vi "X10468 SLM Make Zernike Modes.vi"(0 "R Array":dbl[][](array[numeric]), 7 "Theta Array":dbl[][](array[numeric]), 11 "Number of Modes":i32) -> (8 "Zernike Array":dbl[][][](array[numeric]))   [LabVIEW 2018]
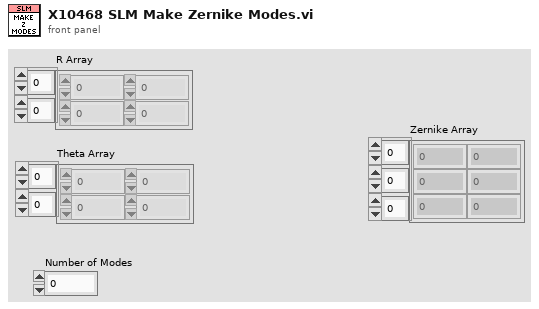
[diagram p1: front panel]
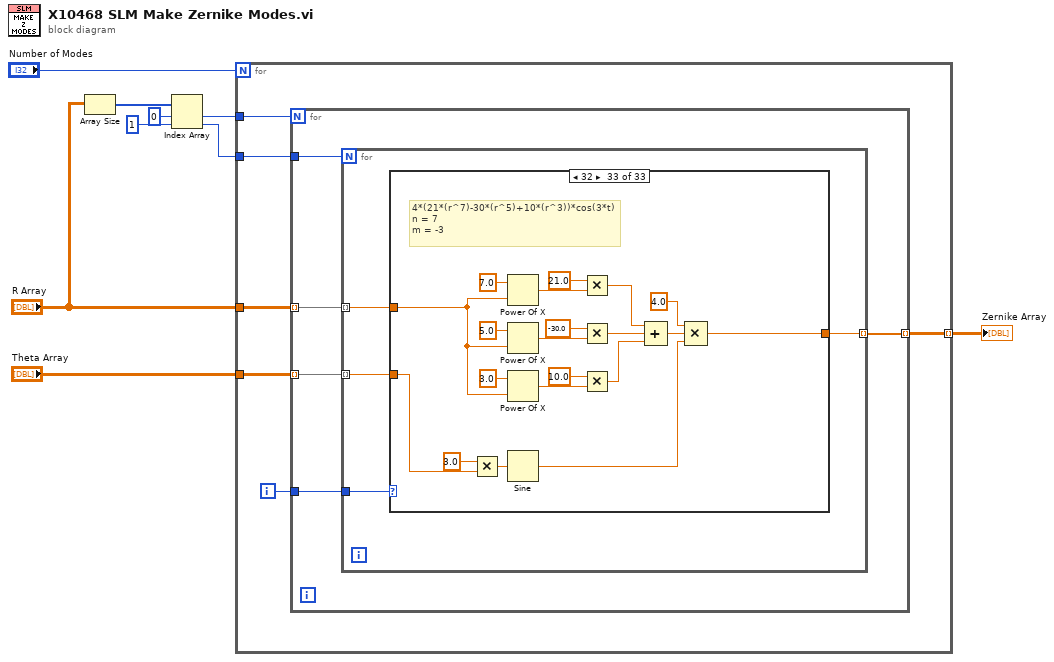
[diagram p0: block diagram]
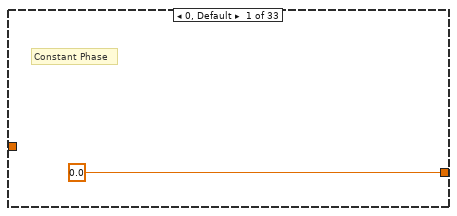
[diagram p2: hidden frame]
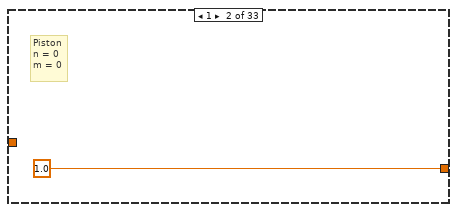
[diagram p3: hidden frame]
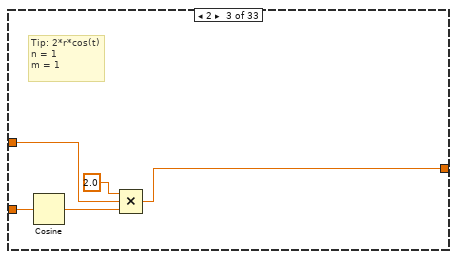
[diagram p4: hidden frame]
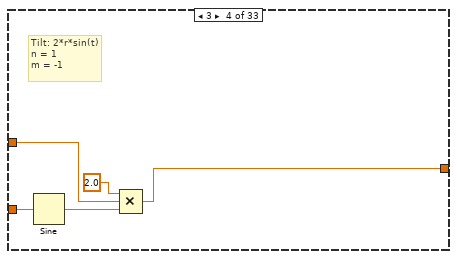
[diagram p5: hidden frame]
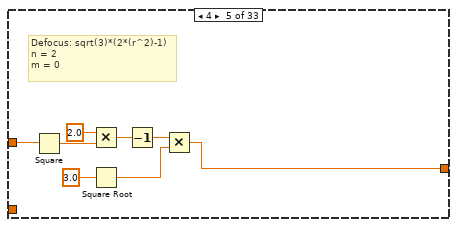
[diagram p6: hidden frame]
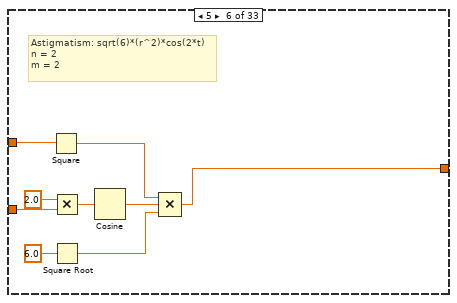
[diagram p7: hidden frame]
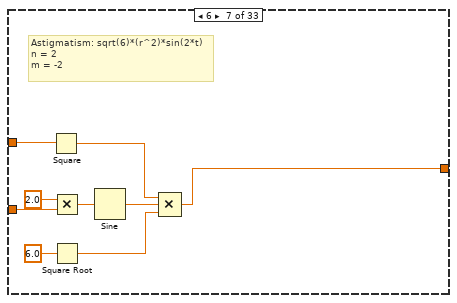
[diagram p8: hidden frame]
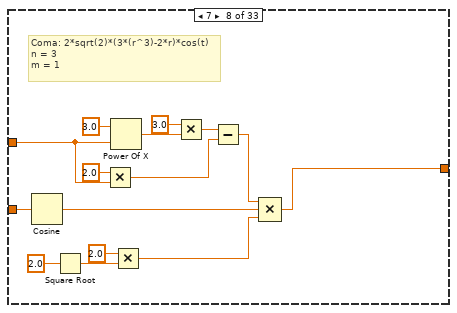
[diagram p9: hidden frame]
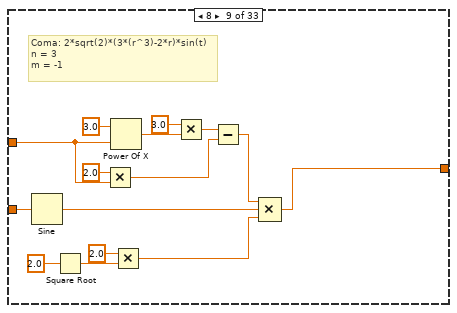
[diagram p10: hidden frame]
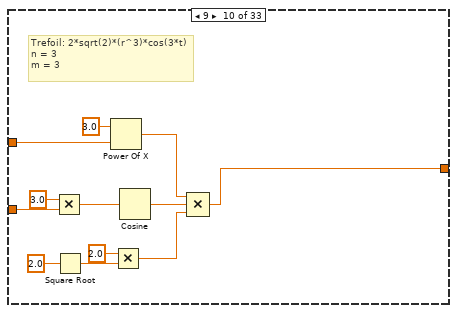
[diagram p11: hidden frame]
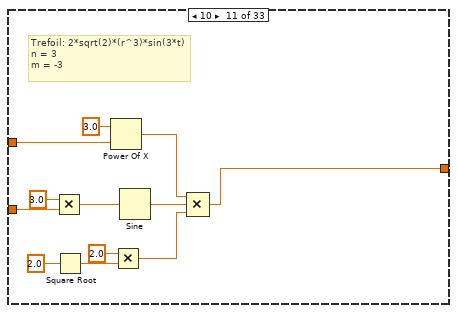
[diagram p12: hidden frame]
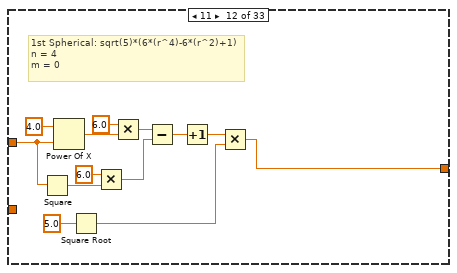
[diagram p13: hidden frame]
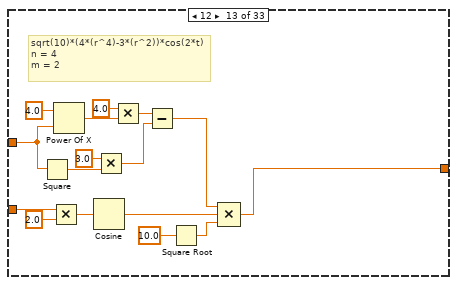
[diagram p14: hidden frame]
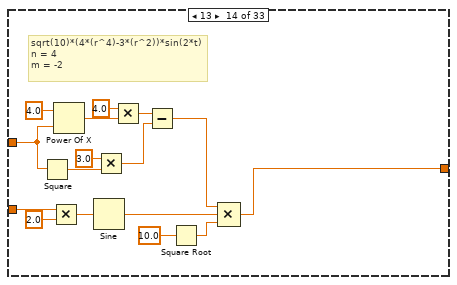
[diagram p15: hidden frame]
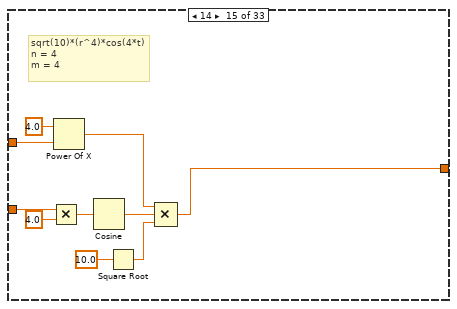
[diagram p16: hidden frame]
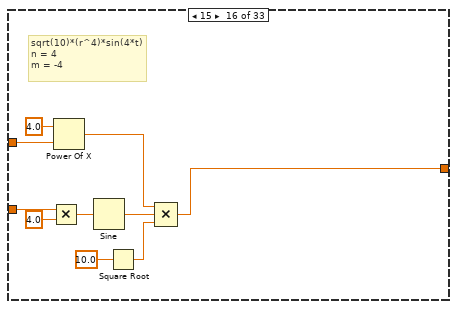
[diagram p17: hidden frame]
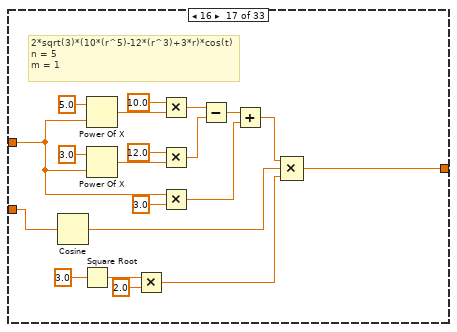
[diagram p18: hidden frame]
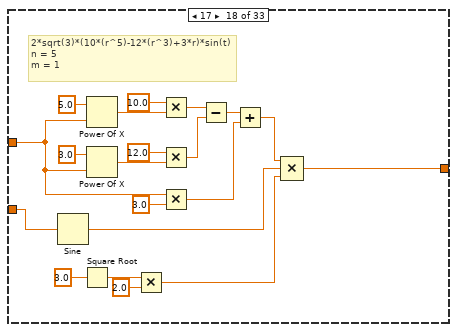
[diagram p19: hidden frame]
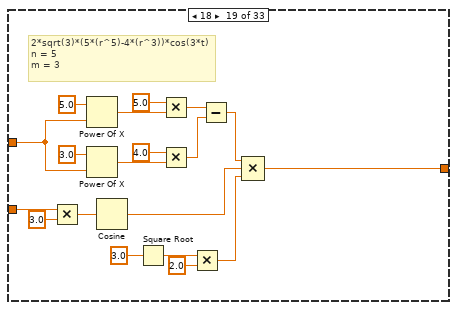
[diagram p20: hidden frame]
diagram:
  n1 = Array Size(array="R Array") -> (size(s)=w8:i32[])
  n2 = Index Array(array=w8, index #1=0 ("index"), index #2=1 ("index")) -> (element #1=w3:i32, element #2=w2:i32)
  n3 = for {
    N: "Number of Modes" -> [_]
    tunnel: "R Array" -> [w11]
    tunnel: "Theta Array" -> [w10]
    tunnel: w3 -> [w15]
    tunnel: w2 -> [w14]
    tunnel: [w12] -> w1 mode=indexing
    i -> [w13]
    n4 = for {
      N: w15 -> [_]
      tunnel: w14 -> [w20]
      tunnel: w13 -> [w19]
      tunnel: [w18] -> w12 mode=indexing
      tunnel: w11 -> [w17] mode=indexing
      tunnel: w10 -> [w16] mode=indexing
      n5 = for {
        N: w20 -> [_]
        tunnel: w19 -> [w24]
        tunnel: [w23] -> w18 mode=indexing
        tunnel: w17 -> [w22] mode=indexing
        tunnel: w16 -> [w21] mode=indexing
        n6 = case shown="32" w24 {
          tunnel: [0.0 1.0 w27 w32 w37 w47 w56 w63 w78 w97 w109 w117 w131 w147 w164 w174 w184 w204 w228 w247 w266 w278 w285 w307 w332 w349 w366 w383 w393 w410 w430 w450 w470] -> w23
          tunnel: w22 -> [_ _ w29 w34 w43 w52 w61 w71 w86 w100 w112 w124 w140 w156 w169 w179 w187 w207 w229 w248 w267 w279 w290 w311 w334 w350 w367 w384 w394 w402 w422 w444 w464]
          tunnel: w21 -> [_ _ w31 w36 _ w51 w60 w76 w91 w95 w107 _ w136 w152 w168 w178 w192 w212 w224 w243 w262 w274 _ w305 w330 w347 w364 w381 w391 w404 w424 w437 w457]
          frame 0, Default {
            # "Constant Phase"
          }
          frame 1 {
            # "Piston\nn = 0\nm = 0"
          }
          frame 2 {
            # "Tip: 2*r*cos(t)\nn = 1\nm = 1"
            n7 = Cosine(x=w31) -> (cos(x)=w30:dbl)
            n8 = Compound Arithmetic op=MULTIPLY(2.0 ("x"), w29, w30) -> (w27:dbl)
          }
          frame 3 {
            # "Tilt: 2*r*sin(t)\nn = 1\nm = -1"
            n9 = Sine(x=w36) -> (sin(x)=w35:dbl)
            n10 = Compound Arithmetic op=MULTIPLY(2.0 ("x"), w34, w35) -> (w32:dbl)
          }
          frame 4 {
            # "Defocus: sqrt(3)*(2*(r^2)-1)\nn = 2\nm = 0"
            n11 = Square(x=w43) -> (x^2=w42:dbl)
            n12 = Multiply(x=2.0, y=w42) -> (x*y=w40:dbl)
            n13 = Square Root(x=3.0) -> (sqrt(x)=w38:dbl)
            n14 = Decrement(x=w40) -> (x-1=w39:dbl)
            n15 = Multiply(x=w39, y=w38) -> (x*y=w37:dbl)
          }
          frame 5 {
            # "Astigmatism: sqrt(6)*(r^2)*cos(2*t)\nn = 2\nm = 2"
            n16 = Square(x=w52) -> (x^2=w48:dbl)
            n17 = Multiply(x=2.0, y=w51) -> (x*y=w49:dbl)
            n18 = Square Root(x=6.0) -> (sqrt(x)=w45:dbl)
            n19 = Cosine(x=w49) -> (cos(x)=w46:dbl)
            n20 = Compound Arithmetic op=MULTIPLY(w48, w46, w45) -> (w47:dbl)
          }
          frame 6 {
            # "Astigmatism: sqrt(6)*(r^2)*sin(2*t)\nn = 2\nm = -2"
            n21 = Square(x=w61) -> (x^2=w57:dbl)
            n22 = Multiply(x=2.0, y=w60) -> (x*y=w58:dbl)
            n23 = Square Root(x=6.0) -> (sqrt(x)=w54:dbl)
            n24 = Sine(x=w58) -> (sin(x)=w55:dbl)
            n25 = Compound Arithmetic op=MULTIPLY(w57, w55, w54) -> (w56:dbl)
          }
          frame 7 {
            # "Coma: 2*sqrt(2)*(3*(r^3)-2*r)*cos(t)\nn = 3\nm = 1"
            n26 = Cosine(x=w76) -> (cos(x)=w65:dbl)
            n27 = Square Root(x=2.0) -> (sqrt(x)=w75:dbl)
            n28 = Multiply(x=2.0, y=w71) -> (x*y=w67:dbl)
            n29 = Power Of X(1:w71, 2:3.0 ("y")) -> (0:w69:dbl)
            n30 = Multiply(x=2.0, y=w75) -> (x*y=w64:dbl)
            n31 = Multiply(x=3.0, y=w69) -> (x*y=w68:dbl)
            n32 = Subtract(x=w68, y=w67) -> (x-y=w66:dbl)
            n33 = Compound Arithmetic op=MULTIPLY(w66, w65, w64) -> (w63:dbl)
          }
          frame 8 {
            # "Coma: 2*sqrt(2)*(3*(r^3)-2*r)*sin(t)\nn = 3\nm = -1"
            n34 = Sine(x=w91) -> (sin(x)=w80:dbl)
            n35 = Square Root(x=2.0) -> (sqrt(x)=w90:dbl)
            n36 = Multiply(x=2.0, y=w86) -> (x*y=w82:dbl)
            n37 = Power Of X(1:w86, 2:3.0 ("y")) -> (0:w84:dbl)
            n38 = Multiply(x=2.0, y=w90) -> (x*y=w79:dbl)
            n39 = Multiply(x=3.0, y=w84) -> (x*y=w83:dbl)
            n40 = Subtract(x=w83, y=w82) -> (x-y=w81:dbl)
            n41 = Compound Arithmetic op=MULTIPLY(w81, w80, w79) -> (w78:dbl)
          }
          frame 9 {
            # "Trefoil: 2*sqrt(2)*(r^3)*cos(3*t)\nn = 3\nm = 3"
            n42 = Multiply(x=3.0, y=w95) -> (x*y=w94:dbl)
            n43 = Square Root(x=2.0) -> (sqrt(x)=w103:dbl)
            n44 = Power Of X(1:w100, 2:3.0 ("y")) -> (0:w93:dbl)
            n45 = Multiply(x=2.0, y=w103) -> (x*y=w98:dbl)
            n46 = Cosine(x=w94) -> (cos(x)=w99:dbl)
            n47 = Compound Arithmetic op=MULTIPLY(w93, w99, w98) -> (w97:dbl)
          }
          frame 10 {
            # "Trefoil: 2*sqrt(2)*(r^3)*sin(3*t)\nn = 3\nm = -3"
            n48 = Multiply(x=3.0, y=w107) -> (x*y=w106:dbl)
            n49 = Square Root(x=2.0) -> (sqrt(x)=w115:dbl)
            n50 = Power Of X(1:w112, 2:3.0 ("y")) -> (0:w105:dbl)
            n51 = Multiply(x=2.0, y=w115) -> (x*y=w110:dbl)
            n52 = Sine(x=w106) -> (sin(x)=w111:dbl)
            n53 = Compound Arithmetic op=MULTIPLY(w105, w111, w110) -> (w109:dbl)
          }
          frame 11 {
            # "1st Spherical: sqrt(5)*(6*(r^4)-6*(r^2)+1)\nn = 4\nm = 0"
            n54 = Square(x=w124) -> (x^2=w123:dbl)
            n55 = Power Of X(1:w124, 2:4.0 ("y")) -> (0:w127:dbl)
            n56 = Square Root(x=5.0) -> (sqrt(x)=w118:dbl)
            n57 = Multiply(x=6.0, y=w123) -> (x*y=w121:dbl)
            n58 = Multiply(x=6.0, y=w127) -> (x*y=w122:dbl)
            n59 = Subtract(x=w122, y=w121) -> (x-y=w120:dbl)
            n60 = Increment(x=w120) -> (x+1=w119:dbl)
            n61 = Multiply(x=w119, y=w118) -> (x*y=w117:dbl)
          }
          frame 12 {
            # "sqrt(10)*(4*(r^4)-3*(r^2))*cos(2*t)\nn = 4\nm = 2"
            n62 = Square(x=w140) -> (x^2=w139:dbl)
            n63 = Multiply(x=w136, y=2.0) -> (x*y=w134:dbl)
            n64 = Power Of X(1:w140, 2:4.0 ("y")) -> (0:w143:dbl)
            n65 = Cosine(x=w134) -> (cos(x)=w130:dbl)
            n66 = Multiply(x=3.0, y=w139) -> (x*y=w137:dbl)
            n67 = Multiply(x=4.0, y=w143) -> (x*y=w138:dbl)
            n68 = Subtract(x=w138, y=w137) -> (x-y=w132:dbl)
            n69 = Square Root(x=10.0) -> (sqrt(x)=w133:dbl)
            n70 = Compound Arithmetic op=MULTIPLY(w132, w130, w133) -> (w131:dbl)
          }
          frame 13 {
            # "sqrt(10)*(4*(r^4)-3*(r^2))*sin(2*t)\nn = 4\nm = -2"
            n71 = Square(x=w156) -> (x^2=w155:dbl)
            n72 = Multiply(x=w152, y=2.0) -> (x*y=w150:dbl)
            n73 = Power Of X(1:w156, 2:4.0 ("y")) -> (0:w159:dbl)
            n74 = Sine(x=w150) -> (sin(x)=w146:dbl)
            n75 = Multiply(x=3.0, y=w155) -> (x*y=w153:dbl)
            n76 = Multiply(x=4.0, y=w159) -> (x*y=w154:dbl)
            n77 = Subtract(x=w154, y=w153) -> (x-y=w148:dbl)
            n78 = Square Root(x=10.0) -> (sqrt(x)=w149:dbl)
            n79 = Compound Arithmetic op=MULTIPLY(w148, w146, w149) -> (w147:dbl)
          }
          frame 14 {
            # "sqrt(10)*(r^4)*cos(4*t)\nn = 4\nm = 4"
            n80 = Multiply(x=w168, y=4.0) -> (x*y=w166:dbl)
            n81 = Power Of X(1:w169, 2:4.0 ("y")) -> (0:w162:dbl)
            n82 = Cosine(x=w166) -> (cos(x)=w163:dbl)
            n83 = Square Root(x=10.0) -> (sqrt(x)=w165:dbl)
            n84 = Compound Arithmetic op=MULTIPLY(w162, w163, w165) -> (w164:dbl)
          }
          frame 15 {
            # "sqrt(10)*(r^4)*sin(4*t)\nn = 4\nm = -4"
            n85 = Multiply(x=w178, y=4.0) -> (x*y=w176:dbl)
            n86 = Power Of X(1:w179, 2:4.0 ("y")) -> (0:w172:dbl)
            n87 = Sine(x=w176) -> (sin(x)=w173:dbl)
            n88 = Square Root(x=10.0) -> (sqrt(x)=w175:dbl)
            n89 = Compound Arithmetic op=MULTIPLY(w172, w173, w175) -> (w174:dbl)
          }
          frame 16 {
            # "2*sqrt(3)*(10*(r^5)-12*(r^3)+3*r)*cos(t)\nn = 5\nm = 1"
            n90 = Cosine(x=w192) -> (cos(x)=w182:dbl)
            n91 = Square Root(x=3.0) -> (sqrt(x)=w194:dbl)
            n92 = Power Of X(1:w187, 2:5.0 ("y")) -> (0:w199:dbl)
            n93 = Power Of X(1:w187, 2:3.0 ("y")) -> (0:w190:dbl)
            n94 = Multiply(x=w194, y=2.0) -> (x*y=w183:dbl)
            n95 = Multiply(x=10.0, y=w199) -> (x*y=w196:dbl)
            n96 = Multiply(x=12.0, y=w190) -> (x*y=w195:dbl)
            n97 = Multiply(x=w187, y=3.0) -> (x*y=w186:dbl)
            n98 = Subtract(x=w196, y=w195) -> (x-y=w189:dbl)
            n99 = Add(x=w189, y=w186) -> (x+y=w185:dbl)
            n100 = Compound Arithmetic op=MULTIPLY(w185, w182, w183) -> (w184:dbl)
          }
          frame 17 {
            # "2*sqrt(3)*(10*(r^5)-12*(r^3)+3*r)*sin(t)\nn = 5\nm = 1"
            n101 = Sine(x=w212) -> (sin(x)=w202:dbl)
            n102 = Square Root(x=3.0) -> (sqrt(x)=w214:dbl)
            n103 = Power Of X(1:w207, 2:5.0 ("y")) -> (0:w219:dbl)
            n104 = Power Of X(1:w207, 2:3.0 ("y")) -> (0:w210:dbl)
            n105 = Multiply(x=w214, y=2.0) -> (x*y=w203:dbl)
            n106 = Multiply(x=10.0, y=w219) -> (x*y=w216:dbl)
            n107 = Multiply(x=12.0, y=w210) -> (x*y=w215:dbl)
            n108 = Multiply(x=w207, y=3.0) -> (x*y=w206:dbl)
            n109 = Subtract(x=w216, y=w215) -> (x-y=w209:dbl)
            n110 = Add(x=w209, y=w206) -> (x+y=w205:dbl)
            n111 = Compound Arithmetic op=MULTIPLY(w205, w202, w203) -> (w204:dbl)
          }
          frame 18 {
            # "2*sqrt(3)*(5*(r^5)-4*(r^3))*cos(3*t)\nn = 5\nm = 3"
            n112 = Multiply(x=w224, y=3.0) -> (x*y=w223:dbl)
            n113 = Power Of X(1:w229, 2:5.0 ("y")) -> (0:w238:dbl)
            n114 = Power Of X(1:w229, 2:3.0 ("y")) -> (0:w230:dbl)
            n115 = Cosine(x=w223) -> (cos(x)=w226:dbl)
            n116 = Square Root(x=3.0) -> (sqrt(x)=w233:dbl)
            n117 = Multiply(x=5.0, y=w238) -> (x*y=w235:dbl)
            n118 = Multiply(x=4.0, y=w230) -> (x*y=w234:dbl)
            n119 = Multiply(x=w233, y=2.0) -> (x*y=w227:dbl)
            n120 = Subtract(x=w235, y=w234) -> (x-y=w222:dbl)
            n121 = Compound Arithmetic op=MULTIPLY(w222, w226, w227) -> (w228:dbl)
          }
          frame 19 {
            # "2*sqrt(3)*(5*(r^5)-4*(r^3))*sin(3*t)\nn = 5\nm = -3"
            n122 = Multiply(x=w243, y=3.0) -> (x*y=w242:dbl)
            n123 = Power Of X(1:w248, 2:5.0 ("y")) -> (0:w257:dbl)
            n124 = Power Of X(1:w248, 2:3.0 ("y")) -> (0:w249:dbl)
            n125 = Sine(x=w242) -> (sin(x)=w245:dbl)
            n126 = Square Root(x=3.0) -> (sqrt(x)=w252:dbl)
            n127 = Multiply(x=5.0, y=w257) -> (x*y=w254:dbl)
            n128 = Multiply(x=4.0, y=w249) -> (x*y=w253:dbl)
            n129 = Multiply(x=w252, y=2.0) -> (x*y=w246:dbl)
            n130 = Subtract(x=w254, y=w253) -> (x-y=w241:dbl)
            n131 = Compound Arithmetic op=MULTIPLY(w241, w245, w246) -> (w247:dbl)
          }
          frame 20 {
            # "2*sqrt(3)*(r^5)*cos(5*t)\nn = 5\nm = 5"
            n132 = Multiply(x=w262, y=5.0) -> (x*y=w261:dbl)
            n133 = Power Of X(1:w267, 2:5.0 ("y")) -> (0:w260:dbl)
            n134 = Cosine(x=w261) -> (cos(x)=w264:dbl)
            n135 = Square Root(x=3.0) -> (sqrt(x)=w269:dbl)
            n136 = Multiply(x=w269, y=2.0) -> (x*y=w265:dbl)
            n137 = Compound Arithmetic op=MULTIPLY(w260, w264, w265) -> (w266:dbl)
          }
          frame 21 {
            # "2*sqrt(3)*(r^5)*sin(5*t)\nn = 5\nm = -5"
            n138 = Multiply(x=w274, y=5.0) -> (x*y=w273:dbl)
            n139 = Power Of X(1:w279, 2:5.0 ("y")) -> (0:w272:dbl)
            n140 = Sine(x=w273) -> (sin(x)=w276:dbl)
            n141 = Square Root(x=3.0) -> (sqrt(x)=w281:dbl)
            n142 = Multiply(x=w281, y=2.0) -> (x*y=w277:dbl)
            n143 = Compound Arithmetic op=MULTIPLY(w272, w276, w277) -> (w278:dbl)
          }
          frame 22 {
            # "sqrt(7)*(20*(r^6)-30*(r^4)+12*r^2-1)\nn = 6\nm = 0"
            n144 = Square(x=w290) -> (x^2=w287:dbl)
            n145 = Power Of X(1:w290, 2:6.0 ("y")) -> (0:w299:dbl)
            n146 = Power Of X(1:w290, 2:4.0 ("y")) -> (0:w293:dbl)
            n147 = Multiply(x=w287, y=12.0) -> (x*y=w288:dbl)
            n148 = Multiply(x=20.0, y=w299) -> (x*y=w296:dbl)
            n149 = Multiply(x=30.0, y=w293) -> (x*y=w295:dbl)
            n150 = Subtract(x=w296, y=w295) -> (x-y=w292:dbl)
            n151 = Add(x=w292, y=w288) -> (x+y=w289:dbl)
            n152 = Square Root(x=7.0) -> (sqrt(x)=w284:dbl)
            n153 = Decrement(x=w289) -> (x-1=w286:dbl)
            n154 = Multiply(x=w286, y=w284) -> (x*y=w285:dbl)
          }
          frame 23 {
            # "sqrt(14)*(15*(r^6)-20*(r^4)+6*r^2)*cos(2*t)\nn = 6\nm = 2"
            n155 = Multiply(x=w305, y=2.0) -> (x*y=w303:dbl)
            n156 = Cosine(x=w303) -> (cos(x)=w302:dbl)
            n157 = Square(x=w311) -> (x^2=w309:dbl)
            n158 = Power Of X(1:w311, 2:6.0 ("y")) -> (0:w320:dbl)
            n159 = Power Of X(1:w311, 2:4.0 ("y")) -> (0:w314:dbl)
            n160 = Multiply(x=w309, y=6.0) -> (x*y=w310:dbl)
            n161 = Multiply(x=15.0, y=w320) -> (x*y=w317:dbl)
            n162 = Multiply(x=20.0, y=w314) -> (x*y=w316:dbl)
            n163 = Subtract(x=w317, y=w316) -> (x-y=w313:dbl)
            n164 = Add(x=w313, y=w310) -> (x+y=w308:dbl)
            n165 = Square Root(x=14.0) -> (sqrt(x)=w306:dbl)
            n166 = Compound Arithmetic op=MULTIPLY(w306, w308, w302) -> (w307:dbl)
          }
          frame 24 {
            # "sqrt(14)*(15*(r^6)-20*(r^4)+6*r^2)*sin(2*t)\nn = 6\nm = -2"
            n167 = Multiply(x=w330, y=2.0) -> (x*y=w328:dbl)
            n168 = Sine(x=w328) -> (sin(x)=w327:dbl)
            n169 = Power Of X(1:w334, 2:6.0 ("y")) -> (0:w340:dbl)
            n170 = Power Of X(1:w334, 2:4.0 ("y")) -> (0:w336:dbl)
            n171 = Square(x=w334) -> (x^2=w333:dbl)
            n172 = Multiply(x=15.0, y=w340) -> (x*y=w323:dbl)
            n173 = Multiply(x=-20.0, y=w336) -> (x*y=w326:dbl)
            n174 = Multiply(x=w333, y=6.0) -> (x*y=w324:dbl)
            n175 = Compound Arithmetic op=ADD(w323, w326, w324) -> (w325:dbl)
            n176 = Square Root(x=14.0) -> (sqrt(x)=w331:dbl)
            n177 = Compound Arithmetic op=MULTIPLY(w331, w325, w327) -> (w332:dbl)
          }
          frame 25 {
            # "sqrt(14)*(6*(r^6)-5*(r^4))*cos(4*t)\nn = 6\nm = 4"
            n178 = Multiply(x=w347, y=4.0) -> (x*y=w345:dbl)
            n179 = Cosine(x=w345) -> (cos(x)=w344:dbl)
            n180 = Power Of X(1:w350, 2:6.0 ("y")) -> (0:w357:dbl)
            n181 = Power Of X(1:w350, 2:4.0 ("y")) -> (0:w351:dbl)
            n182 = Multiply(x=6.0, y=w357) -> (x*y=w354:dbl)
            n183 = Multiply(x=5.0, y=w351) -> (x*y=w353:dbl)
            n184 = Subtract(x=w354, y=w353) -> (x-y=w343:dbl)
            n185 = Square Root(x=14.0) -> (sqrt(x)=w348:dbl)
            n186 = Compound Arithmetic op=MULTIPLY(w348, w343, w344) -> (w349:dbl)
          }
          frame 26 {
            # "sqrt(14)*(6*(r^6)-5*(r^4))*sin(4*t)\nn = 6\nm = -4"
            n187 = Multiply(x=w364, y=4.0) -> (x*y=w362:dbl)
            n188 = Sine(x=w362) -> (sin(x)=w361:dbl)
            n189 = Power Of X(1:w367, 2:6.0 ("y")) -> (0:w374:dbl)
            n190 = Power Of X(1:w367, 2:4.0 ("y")) -> (0:w368:dbl)
            n191 = Multiply(x=6.0, y=w374) -> (x*y=w371:dbl)
            n192 = Multiply(x=5.0, y=w368) -> (x*y=w370:dbl)
            n193 = Subtract(x=w371, y=w370) -> (x-y=w360:dbl)
            n194 = Square Root(x=14.0) -> (sqrt(x)=w365:dbl)
            n195 = Compound Arithmetic op=MULTIPLY(w365, w360, w361) -> (w366:dbl)
          }
          frame 27 {
            # "sqrt(14)*(r^6)*cos(6*t)\nn = 6\nm = 6"
            n196 = Multiply(x=w381, y=6.0) -> (x*y=w379:dbl)
            n197 = Power Of X(1:w384, 2:6.0 ("y")) -> (0:w377:dbl)
            n198 = Cosine(x=w379) -> (cos(x)=w378:dbl)
            n199 = Square Root(x=14.0) -> (sqrt(x)=w382:dbl)
            n200 = Compound Arithmetic op=MULTIPLY(w382, w377, w378) -> (w383:dbl)
          }
          frame 28 {
            # "sqrt(14)*(r^6)*sin(6*t)\nn = 6\nm = 6"
            n201 = Multiply(x=w391, y=6.0) -> (x*y=w389:dbl)
            n202 = Power Of X(1:w394, 2:6.0 ("y")) -> (0:w387:dbl)
            n203 = Sine(x=w389) -> (sin(x)=w388:dbl)
            n204 = Square Root(x=14.0) -> (sqrt(x)=w392:dbl)
            n205 = Compound Arithmetic op=MULTIPLY(w392, w387, w388) -> (w393:dbl)
          }
          frame 29 {
            # "4*(35*(r^7)-60*(r^5)+30*(r^3)-4*r)*cos(t)\nn = 7\nm = 1"
            n206 = Cosine(x=w404) -> (cos(x)=w409:dbl)
            n207 = Power Of X(1:w402, 2:7.0 ("y")) -> (0:w415:dbl)
            n208 = Power Of X(1:w402, 2:5.0 ("y")) -> (0:w411:dbl)
            n209 = Power Of X(1:w402, 2:3.0 ("y")) -> (0:w407:dbl)
            n210 = Multiply(x=35.0, y=w415) -> (x*y=w401:dbl)
            n211 = Multiply(x=-60.0, y=w411) -> (x*y=w398:dbl)
            n212 = Multiply(x=30.0, y=w407) -> (x*y=w399:dbl)
            n213 = Multiply(x=-4.0, y=w402) -> (x*y=w397:dbl)
            n214 = Compound Arithmetic op=ADD(w401, w398, w399, w397) -> (w400:dbl)
            n215 = Compound Arithmetic op=MULTIPLY(4.0 ("x"), w400, w409) -> (w410:dbl)
          }
          frame 30 {
            # "4*(35*(r^7)-60*(r^5)+30*(r^3)-4*r)*sin(t)\nn = 7\nm = -1"
            n216 = Sine(x=w424) -> (sin(x)=w429:dbl)
            n217 = Power Of X(1:w422, 2:7.0 ("y")) -> (0:w435:dbl)
            n218 = Power Of X(1:w422, 2:5.0 ("y")) -> (0:w431:dbl)
            n219 = Power Of X(1:w422, 2:3.0 ("y")) -> (0:w427:dbl)
            n220 = Multiply(x=35.0, y=w435) -> (x*y=w421:dbl)
            n221 = Multiply(x=-60.0, y=w431) -> (x*y=w418:dbl)
            n222 = Multiply(x=30.0, y=w427) -> (x*y=w419:dbl)
            n223 = Multiply(x=-4.0, y=w422) -> (x*y=w417:dbl)
            n224 = Compound Arithmetic op=ADD(w421, w418, w419, w417) -> (w420:dbl)
            n225 = Compound Arithmetic op=MULTIPLY(4.0 ("x"), w420, w429) -> (w430:dbl)
          }
          frame 31 {
            # "4*(21*(r^7)-30*(r^5)+10*(r^3))*cos(3*t)\nn = 7\nm = 3"
            n226 = Multiply(x=3.0, y=w437) -> (x*y=w438:dbl)
            n227 = Power Of X(1:w444, 2:7.0 ("y")) -> (0:w455:dbl)
            n228 = Power Of X(1:w444, 2:5.0 ("y")) -> (0:w451:dbl)
            n229 = Power Of X(1:w444, 2:3.0 ("y")) -> (0:w447:dbl)
            n230 = Cosine(x=w438) -> (cos(x)=w449:dbl)
            n231 = Multiply(x=21.0, y=w455) -> (x*y=w443:dbl)
            n232 = Multiply(x=-30.0, y=w451) -> (x*y=w440:dbl)
            n233 = Multiply(x=10.0, y=w447) -> (x*y=w441:dbl)
            n234 = Compound Arithmetic op=ADD(w443, w440, w441) -> (w442:dbl)
            n235 = Compound Arithmetic op=MULTIPLY(4.0 ("x"), w442, w449) -> (w450:dbl)
          }
          frame 32 {
            # "4*(21*(r^7)-30*(r^5)+10*(r^3))*cos(3*t)\nn = 7\nm = -3"
            n236 = Multiply(x=3.0, y=w457) -> (x*y=w458:dbl)
            n237 = Power Of X(1:w464, 2:7.0 ("y")) -> (0:w475:dbl)
            n238 = Power Of X(1:w464, 2:5.0 ("y")) -> (0:w471:dbl)
            n239 = Power Of X(1:w464, 2:3.0 ("y")) -> (0:w467:dbl)
            n240 = Sine(x=w458) -> (sin(x)=w469:dbl)
            n241 = Multiply(x=21.0, y=w475) -> (x*y=w463:dbl)
            n242 = Multiply(x=-30.0, y=w471) -> (x*y=w460:dbl)
            n243 = Multiply(x=10.0, y=w467) -> (x*y=w461:dbl)
            n244 = Compound Arithmetic op=ADD(w463, w460, w461) -> (w462:dbl)
            n245 = Compound Arithmetic op=MULTIPLY(4.0 ("x"), w462, w469) -> (w470:dbl)
          }
        }
      }
    }
  }
  "Zernike Array" <- w1
